vi "Initialize.vi"(8 "error in":errorcluster, 11 "menu reference":refnum<k9>) -> (0 "error out":errorcluster, 3 "History":refnum<class "History.lvclass">)   [LabVIEW 2020, in "lv_icon.lvlib" / "History.lvlib" / "History.lvclass"]
doc: "Initializes the history class."
uses:
  History.lvclass
  History.lvclass/History.ctl
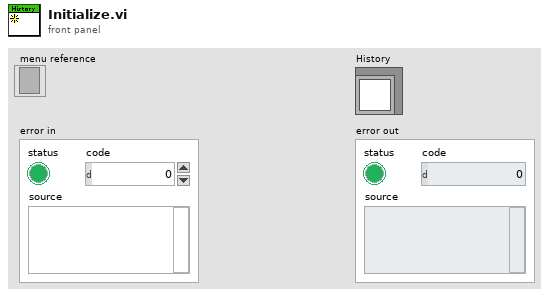
[diagram p1: front panel]
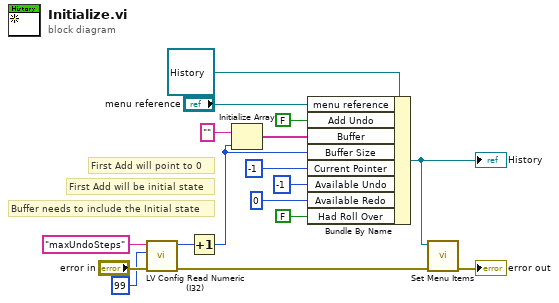
[diagram p0: block diagram]
diagram:
  # "First Add will be initial state"
  # "First Add will point to 0"
  # "Buffer needs to include the Initial state"
  n1 = call <resource>:"LV Config Read Numeric (I32).vi"("error in"="error in", "default value"=99, "key"="maxUndoSteps") -> ("error out"=w16:errorcluster, "value"=w12:i32)  [unwired: 2 in, 1 out]
  n2 = Increment(x=w12) -> (x+1=w8:i32)
  n3 = Initialize Array("", w8) -> (w7:string[])
  n4 = Bundle By Name(cluster=refnum<class "History.lvclass"> refnum ("lv_icon.lvlib:History.lvlib:History.lvclass"), "menu reference"="menu reference", "Add Undo"=FALSE, "Buffer"=w7, "Buffer Size"=w8, "Current Pointer"=-1, "Available Undo"=-1, "Available Redo"=0, "Had Roll Over"=FALSE) -> (w1:refnum<class "History.lvclass">)
  "History" <- w1
  n5 = call "Set Menu Items.vi"("error in"=w16, "History"=w1) -> ("error out"=→"error out":errorcluster)  [unwired: 9 in]
